vi "GPIB Send.vi"(0 "GPIB Setup":cluster{"GPIB address":i16, "GPIB bus":i16}={"GPIB address"=1, "GPIB bus"=0}, 1 "Input command":string, 2 "error in":T1) -> (3 "Return string":string, 4 "Bytes sent":i32, 5 "Spoll byte (bits 7 thru 1)":i16 format="%.0b", 6 "error out":T1)   [LabVIEW 2016]
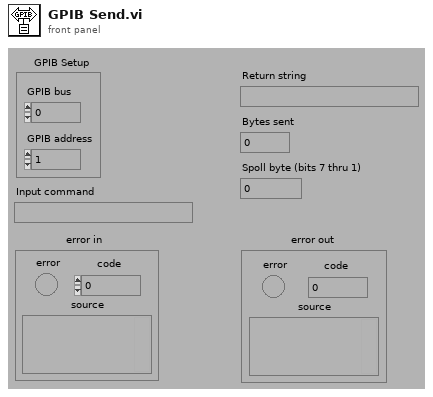
[diagram p1: front panel]
types:
  T1 = cluster{"error":bool, "code":i32, "source":string}
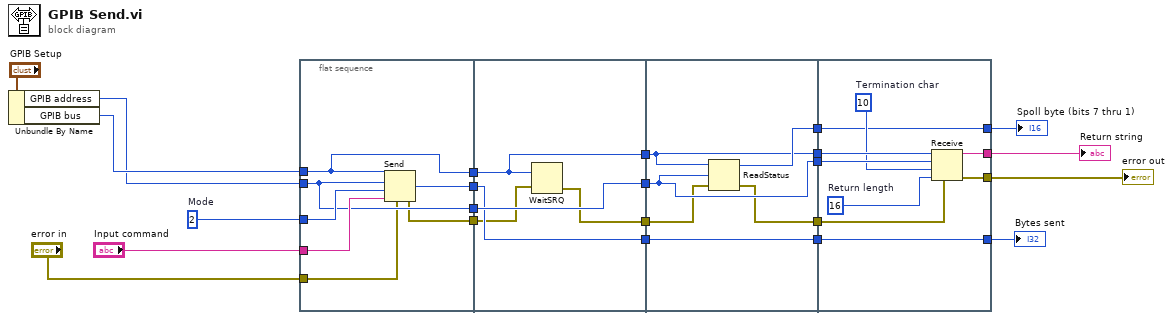
[diagram p0: block diagram]
diagram:
  w23 = u8 2  # Mode
  n1 = Unbundle By Name("GPIB Setup") -> ("GPIB address"=w18:i16, "GPIB bus"=w19:i16)
  n2 = flat-sequence {
    tunnel: w18 -> [w27]
    tunnel: [w27] -> w17
    tunnel: "Input command" -> [w30]
    tunnel: w19 -> [w26]
    tunnel: [w26] -> w16
    tunnel: w23 -> [w29]
    tunnel: [w28] -> w15
    tunnel: [w25] -> w7
    tunnel: "error in" -> [w24]
    tunnel: w17 -> [w35]
    tunnel: [w35] -> w14
    tunnel: w16 -> [w34]
    tunnel: [w34] -> w13
    tunnel: w15 -> [w33]
    tunnel: [w33] -> w12
    tunnel: w7 -> [w32]
    tunnel: [w31] -> w6
    tunnel: w14 -> [w40]
    tunnel: [w40] -> w11
    tunnel: w13 -> [w39]
    tunnel: [w39] -> w10
    tunnel: w12 -> [w38]
    tunnel: [w38] -> w9
    tunnel: [w41] -> w8
    tunnel: w6 -> [w37]
    tunnel: [w36] -> w5
    tunnel: w11 -> [w49]
    tunnel: w10 -> [w50]
    tunnel: [w46] -> w2
    tunnel: [w45] -> w21
    tunnel: w9 -> [w45]
    tunnel: [w44] -> w22
    tunnel: w8 -> [w44]
    tunnel: w5 -> [w43]
    tunnel: [w42] -> w1
    frame #0 {
      n3 = Send(0:w26, 2:w27, 3:w29, 4:w24, 5:w30) -> (7:w28:i32, 8:w25:errorcluster)  [unwired: 1 out]
    }
    frame #1 {
      n4 = WaitSRQ(0:w34, 1:w32) -> (4:w31:errorcluster)  [unwired: 2 out]
    }
    frame #2 {
      n5 = ReadStatus(3:w37, 4:w40, 5:w39) -> (0:w36:errorcluster, 2:w41:i16)  [unwired: 1 out]
    }
    frame #3 {
      w47 = 16  # Return length
      w48 = u16 10  # Termination char
      n6 = Receive(4:w43, 6:w47, 7:w48, 8:w49, 9:w50) -> (0:w42:errorcluster, 3:w46:string)  [unwired: 2 out]
    }
  }
  "Bytes sent" <- w21
  "Spoll byte (bits 7 thru 1)" <- w22
  "Return string" <- w2
  "error out" <- w1
